vi "bead_dropper.vi"() -> ()   [LabVIEW 2018]
uses:
  <vilib>/Instr/_visa.llb/VISA Open Access Mode.ctl
  <instrlib>/Agilent 33XXX Series/Agilent 33XXX Series.lvlib
panel:
  in  "seconds between steps":u32=5
  out "Last Voltage":dbl=13.95
  in  "stop":bool
  in  "Stop  Frequency (kHz)":dbl=700.0 format="%#.6g"
  in  "Start Frequency (kHz)":dbl=100.0 format="%#.6g"
  in  "Sweep Time (s)":dbl=0.1 format="%#.6g"
  in  "Step size (V)":dbl=0.05
  in  "Start Voltage (V)":dbl=13.7
  in  "Number of steps":i32=30
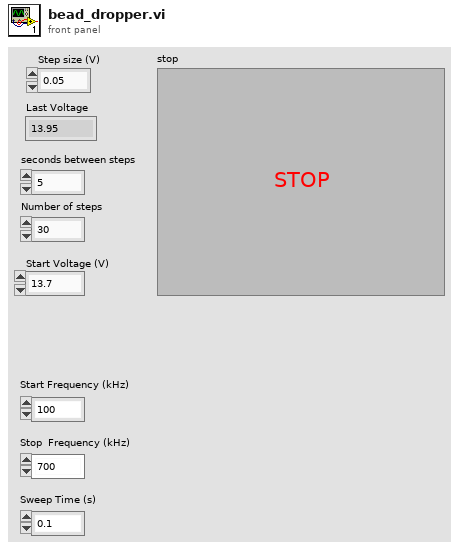
[diagram p1: front panel]
types:
  T1 = typedef "VISA Open Access Mode.ctl" = u32
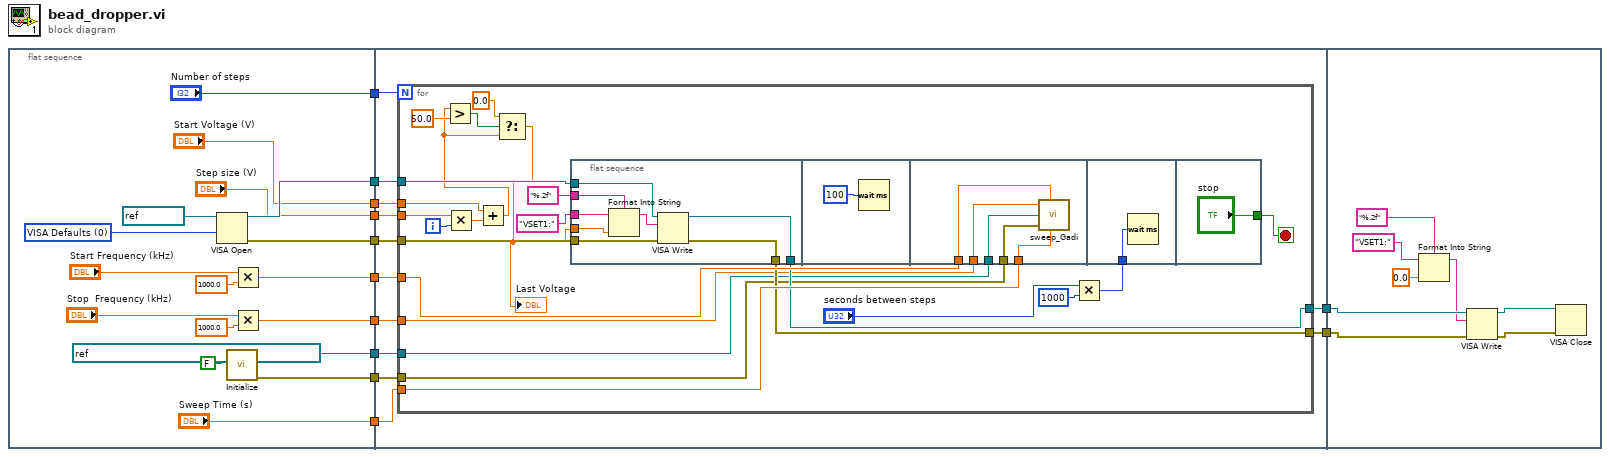
[diagram p0: block diagram]
diagram:
  n1 = flat-sequence {
    tunnel: ["Number of steps"] -> w12
    tunnel: [w25] -> w11
    tunnel: [w24] -> w10
    tunnel: [w19] -> w9
    tunnel: [w18] -> w8
    tunnel: ["Sweep Time (s)"] -> w7
    tunnel: ["Start Voltage (V)"] -> w6
    tunnel: ["Step size (V)"] -> w5
    tunnel: [w14] -> w2
    tunnel: [w13] -> w1
    tunnel: w12 -> [w42]
    tunnel: w11 -> [w41]
    tunnel: w10 -> [w40]
    tunnel: w9 -> [w39]
    tunnel: w8 -> [w38]
    tunnel: w7 -> [w37]
    tunnel: w6 -> [w36]
    tunnel: w5 -> [w35]
    tunnel: [w34] -> w4
    tunnel: [w33] -> w3
    tunnel: w2 -> [w32]
    tunnel: w1 -> [w31]
    tunnel: w4 -> [w90]
    tunnel: w3 -> [w88]
    frame #0 {
      w27 = T1 0 items=["VISA Defaults"=0, "Exclusive Lock"=1, "Load Configured Settings"=4] ("Access Mode")
      n2 = VISA Open(access mode=w27, VISA resource name=refnum<visa-resource-name> "COM5") -> (VISA resource name=w25:refnum<visa-resource-name>, error out=w24:errorcluster)  [unwired: 3 in]
      n3 = call <instrlib>:"Initialize.vi"("ID Query (True)"=FALSE, "VISA resource name"=refnum<visa-resource-name> "USB0::0x0957::0x2707::MY57301756::INSTR") -> ("error out"=w14:errorcluster, "VISA resource name out"=w13:refnum<visa-resource-name>)  [unwired: 8 in]
      n4 = Multiply(x="Start Frequency (kHz)", y=1000.0) -> (x*y=w18:dbl)
      n5 = Multiply(x="Stop  Frequency (kHz)", y=1000.0) -> (x*y=w19:dbl)
    }
    frame #1 {
      n6 = for {
        N: w42 -> [_]
        tunnel: w36 -> [w66]
        tunnel: w35 -> [w65]
        tunnel: w38 -> [w59]
        tunnel: w37 -> [w60]
        tunnel: w41 -> [w58]
        tunnel: [w57] -> w33
        tunnel: w40 -> [w56]
        tunnel: [w55] -> w34
        tunnel: w39 -> [w50]
        tunnel: w32 -> [w49]
        tunnel: w31 -> [w48]
        i -> [w64]
        stop <- w51 stop-if-true
        n7 = Multiply(x=w65, y=w64) -> (x*y=w63:dbl)
        n8 = Add(x=w66, y=w63) -> (x+y=w44:dbl)
        n9 = Greater?(x=w44, y=50.0) -> (0:w47:bool)
        n10 = Select(t=0.0, s=w47, f=w44) -> (s? t:f=w43:dbl)
        "Last Voltage" <- w43
        n11 = flat-sequence {
          tunnel: w43 -> [w74]
          tunnel: "VSET1:" ("write buffer") -> [w73]
          tunnel: "%.2f" ("format string") -> [w72]
          tunnel: w58 -> [w71]
          tunnel: [w70] -> w57
          tunnel: w56 -> [w69]
          tunnel: [w68] -> w55
          tunnel: w60 -> [w76]
          tunnel: w59 -> [w77]
          tunnel: w50 -> [w78]
          tunnel: w49 -> [w80]
          tunnel: w48 -> [w79]
          tunnel: w52 -> [w81]
          tunnel: ["stop"] -> w51
          frame #0 {
            n12 = Format Into String(format string=w72, initial string=w73, w74) -> (resulting string=w67:string)  [unwired: 1 in, 1 out]
            n13 = VISA Write(VISA resource name=w71, write buffer=w67, error in (no error)=w69) -> (VISA resource name out=w70:refnum<visa-resource-name>, error out=w68:errorcluster)  [unwired: 1 out]
          }
          frame #1 {
            n14 = Wait (ms)(milliseconds to wait=u32 100) -> ()  [unwired: 1 out]
          }
          frame #2 {
            n15 = call "sweep_Gadi.vi"("Stop  Frequency (1000.0 Hz)"=w78, "Start Frequency (100.0 Hz)"=w77, "VISA resource name in"=w79, "error in (no error)"=w80, "Sweep Time (1.00 s)"=w76) -> ()  [unwired: 5 in]
          }
          frame #3 {
            n16 = Wait (ms)(milliseconds to wait=w81) -> ()  [unwired: 1 out]
          }
          frame #4 {
          }
        }
        n17 = Multiply(x="seconds between steps", y=u32 1000) -> (x*y=w52:u32)
      }
    }
    frame #2 {
      n18 = Format Into String(format string="%.2f", initial string="VSET1:" ("write buffer"), 0.0 ("input 1")) -> (resulting string=w84:string)  [unwired: 1 in, 1 out]
      n19 = VISA Write(VISA resource name=w88, write buffer=w84, error in (no error)=w90) -> (VISA resource name out=w87:refnum<visa-resource-name>, error out=w89:errorcluster)  [unwired: 1 out]
      n20 = VISA Close(VISA resource name=w87, error in (no error)=w89) -> ()  [unwired: 1 out]
    }
  }
